vi "Dashboat.vi"() -> ()   [LabVIEW 2019]
uses:
  <vilib>/Utility/miscctls.llb/LVPositionTypeDef.ctl
  Documents/2468 Team Appreciate/2019/Software/2019 Deep Space Dashboard/Front Camera Variables.vi
panel:
  out "Bottom Camera Image":T1(plugin-control)
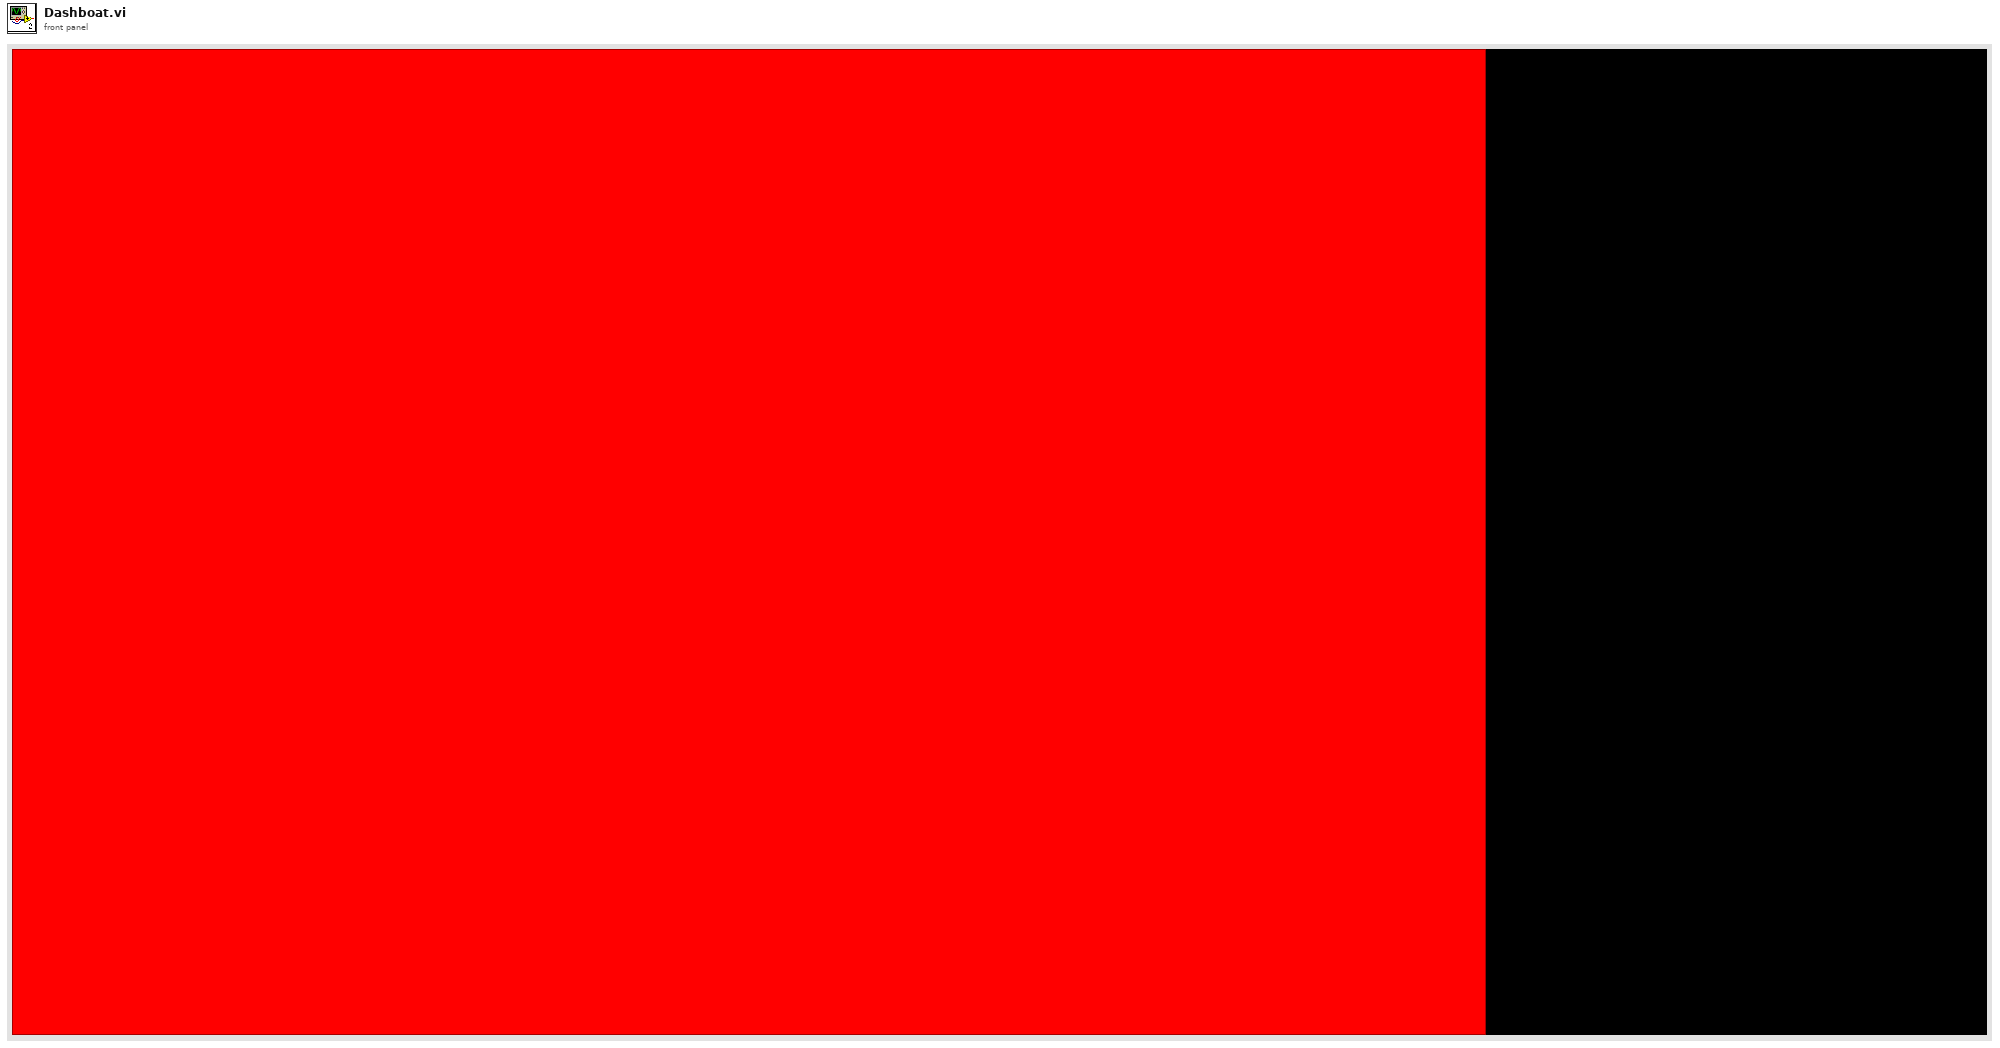
[diagram p1: front panel]
types:
  T1 = typedef "IMAQ Image.ctl" = refnum<image>
  T2 = typedef "LVPositionTypeDef.ctl" = cluster{"Left":i32, "Top":i32}
  T3 = cluster{"Global Rectangle":i32[], "Contours":cluster{"Contour Type":u32, "ROI Type":u32, "Points":i32[]}[]}
  T4 = typedef "LVRectTypeDef.ctl" = cluster{"Left":i16, "Top":i16, "Right":i16, "Bottom":i16}
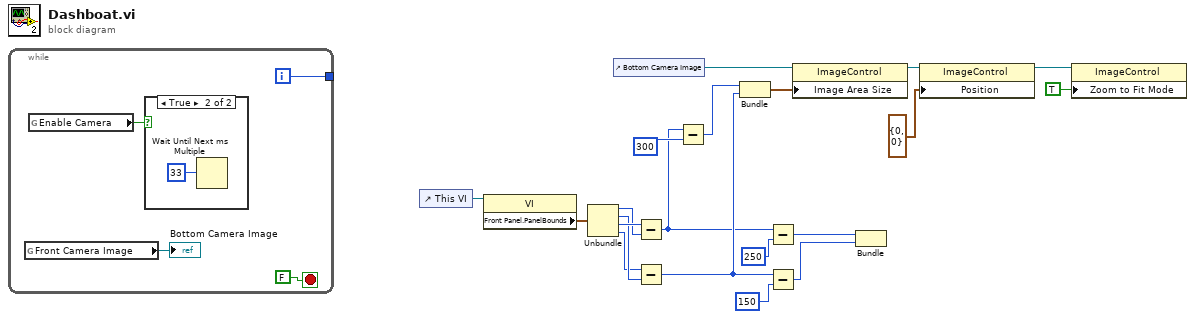
[diagram p0: block diagram]
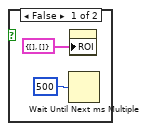
[diagram p2: hidden frame]
diagram:
  n1 = while {
    tunnel: [w23] -> _
    i -> [w23]
    stop <- FALSE stop-if-true
    n2 = global read "Front Camera Variables.vi" "Front Camera Image"() -> (→"Bottom Camera Image":T1)
    n3 = global read "Front Camera Variables.vi" "Enable Camera"() -> (w21:bool)
    n4 = case shown="True" w21 {
      frame False {
        n5 = Wait Until Next ms Multiple(millisecond multiple=u32 500) -> ()  [unwired: 1 out]
        n6 = property on="Bottom Camera Image" class="ImageControl"("ROI"=T3 {"Global Rectangle"=[], "Contours"=[]}) -> ()  [unwired: 2 in, 2 out]
      }
      frame True {
        n7 = Wait Until Next ms Multiple(millisecond multiple=u32 33) -> ()  [unwired: 1 out]
      }
    }
  }
  n8 = control-ref of="This VI"() -> (w19:refnum<vi>)
  n9 = property class="VI"(reference=w19) -> ("Front Panel.PanelBounds"=w18:T4)  [unwired: 1 in, 2 out]
  n10 = Unbundle(w18) -> ("Left"=w16:i16, "Top"=w11:i16, "Right"=w17:i16, "Bottom"=w9:i16)
  n11 = control-ref of="Bottom Camera Image"() -> (w20:refnum<vi>)
  n12 = Subtract(x=w17, y=w16) -> (x-y=w2:i16)
  n13 = Subtract(x=w9, y=w11) -> (x-y=w8:i16)
  n14 = Subtract(x=w2, y=i16 300) -> (x-y=w1:i16)
  n15 = Bundle(w1, w8) -> (w10:cluster{i16, i16})  [unwired: 1 in]
  n16 = Subtract(x=w2, y=i16 250) -> (x-y=w4:i16)
  n17 = Subtract(x=w8, y=i16 150) -> (x-y=w5:i16)
  n18 = property class="ImageControl"(reference=w20, "Image Area Size"=w10) -> (reference out=w14:refnum<vi>)  [unwired: 1 in, 1 out]
  n19 = Bundle(w4, w5) -> ()  [unwired: 1 in, 1 out]
  n20 = property class="ImageControl"(reference=w14, "Position"=T2 {"Left"=0, "Top"=0}) -> (reference out=w13:refnum<vi>)  [unwired: 1 in, 1 out]
  n21 = property class="ImageControl"(reference=w13, "Zoom to Fit Mode"=TRUE) -> ()  [unwired: 1 in, 2 out]
